vi "Fetch Acquired Data.vi"   [LabVIEW 2012]
uses:
  <userlib>/FlexRIO Host Library/FlexRIO Host Library (User).lvlib
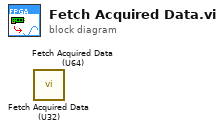
[diagram p0: block diagram]
diagram:
  n1 = call <userlib>:"Fetch Acquired Data (U32).vi"() -> ()  [unwired: 8 in, 4 out]
  n2 = call <userlib>:"Fetch Acquired Data (U64).vi"() -> ()  [unwired: 8 in, 4 out]
